vi "mod_Calculate Correction.vi"   [LabVIEW 2020, in "niAMT.lvlib"]
doc: "Calculates a correction to compensate a spectrum for the amplitude response of signal conditioners and digitizers. Use your instrument drivers to determine the values you enter in the <B>calibration</B> cluster."
uses:
  <vilib>/addons/Modulation/niAMT.lvlib
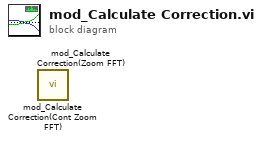
[diagram p0: block diagram]
diagram:
  n1 = call <vilib>:"mod_Calculate Correction(Cont Zoom FFT).vi"() -> ()  [unwired: 10 in, 2 out]
  n2 = call <vilib>:"mod_Calculate Correction(Zoom FFT).vi"() -> ()  [unwired: 10 in, 2 out]
